vi "Test Coffee Shop Remove Customer Broadcast Name.vi"(8 "error in (no error)":errorcluster, 11 "Coffee Shop Test In":refnum<class "Coffee Shop Test.lvclass">) -> (0 "error out":errorcluster, 3 "Coffee Shop Test Out":refnum<class "Coffee Shop Test.lvclass">)   [LabVIEW 2020, in "Coffee Shop Test.lvclass"]
uses:
  Coffee Shop Test.lvclass
  Coffee Shop/Coffee Shop.lvclass
  <vilib>/Asteme/Triarc Framework/Process/Process.lvclass
  C:/Program Files (x86)/National Instruments/LabVIEW 2020/vi.lib/Asteme/Triarc Framework/Application/Application.lvclass
  C:/Program Files (x86)/National Instruments/LabVIEW 2020/vi.lib/Asteme/Triarc Framework/Process/Process.lvclass
  C:/Program Files (x86)/National Instruments/LabVIEW 2020/vi.lib/Asteme/Triarc Framework/Base/Base.lvclass
  C:/Program Files (x86)/National Instruments/LabVIEW 2020/vi.lib/Asteme/Triarc Framework/Error Handler Interface/Error Handler Interface.lvclass
  C:/Program Files (x86)/National Instruments/LabVIEW 2020/vi.lib/Asteme/Triarc Framework/Logging/Logging.lvclass
  C:/Users/anton/Documents/GitHub/Triarc-Examples/Coffee Shop/Coffee Shop/Coffee Shop.lvclass
  <vilib>/Asteme/Triarc Framework Test Suite/Support/Event Helpers/Event Helpers.lvlib
  <vilib>/Asteme/LUnit/Test Case.lvclass
  C:/Program Files (x86)/National Instruments/LabVIEW 2020/vi.lib/Asteme/Triarc Framework Test Suite/Application Test/Application Test.lvclass
  C:/Program Files (x86)/National Instruments/LabVIEW 2020/vi.lib/Asteme/Triarc Framework Test Suite/Process Test/Process Test.lvclass
  C:/Program Files (x86)/National Instruments/LabVIEW 2020/vi.lib/Asteme/Triarc Framework Test Suite/Base Class Test/Base Test.lvclass
  C:/Program Files (x86)/National Instruments/LabVIEW 2020/vi.lib/Asteme/LUnit/Test Case.lvclass
  C:/Users/anton/Documents/GitHub/Triarc-Examples/Coffee Shop/Coffee Shop Test/Coffee Shop Test.lvclass
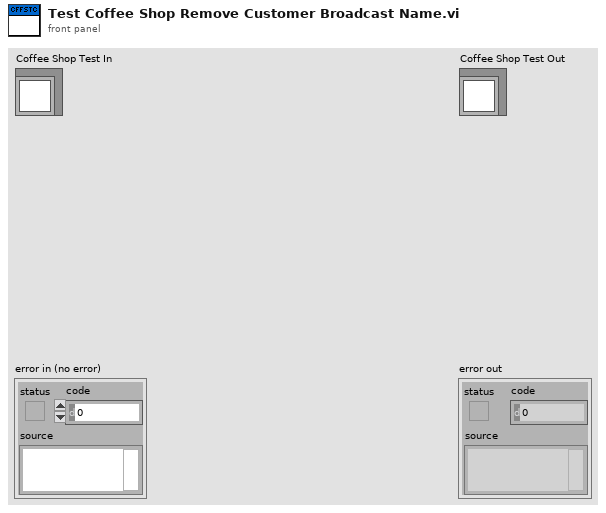
[diagram p1: front panel]
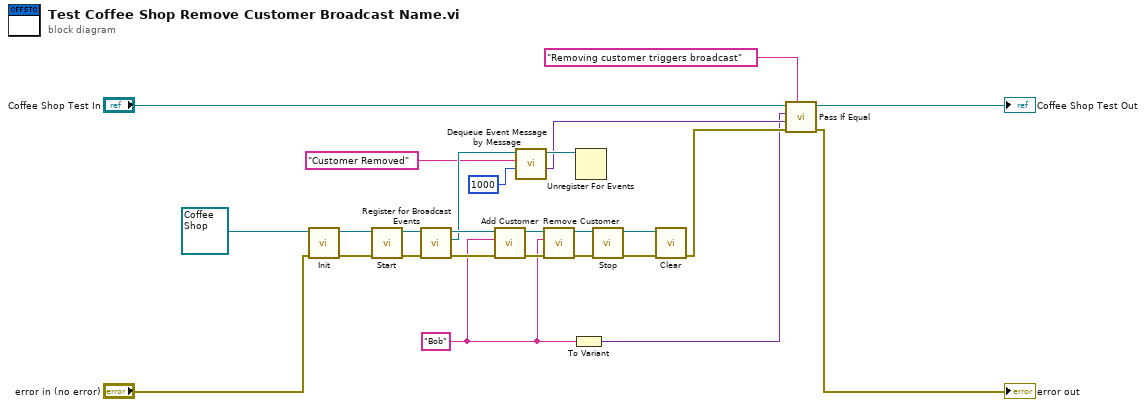
[diagram p0: block diagram]
diagram:
  w1 = "Bob" ("Name")
  n1 = call-dynamic "Init.vi"("error in (no error)"="error in (no error)", "Process In"=refnum<class "Coffee Shop.lvclass"> refnum ("Coffee Shop.lvclass")) -> ("error out"=w24:errorcluster, "Process Out"=w25:refnum<class "Coffee Shop.lvclass">)  [unwired: 8 in]
  n2 = call <vilib>:"Start.vi"("error in (no error)"=w24, "Process In"=w25) -> ("error out"=w23:errorcluster, "Process Out"=w17:refnum<class "Coffee Shop.lvclass">)  [unwired: 8 in]
  n3 = call <vilib>:"Register for Broadcast Events.vi"("error in (no error)"=w23, "Process In"=w17) -> ("error out"=w18:errorcluster, "Event Registration Refnum Out"=w15:refnum<event-registration>, "Process Out"=w16:refnum<class "Coffee Shop.lvclass">)  [unwired: 7 in]
  n4 = call "Add Customer.vi"("error in (no error)"=w18, "Name"=w1, "Coffee Shop in"=w16) -> ("error out"=w19:errorcluster, "Coffee Shop out"=w3:refnum<class "Coffee Shop.lvclass">)  [unwired: 7 in]
  n5 = call <vilib>:"Dequeue Event Message by Message.vi"("Timeout (-1)"=1000, "Message"="Customer Removed", "Event Registration Refnum"=w15) -> ("Message Data"=w6:variant, "Event Registration Refnum Out"=w13:refnum<event-registration>)  [unwired: 4 in, 3 out]
  n6 = call "Remove Customer.vi"("error in (no error)"=w19, "Name"=w1, "Coffee Shop In"=w3) -> ("error out"=w4:errorcluster, "Coffee Shop Out"=w2:refnum<class "Coffee Shop.lvclass">)  [unwired: 7 in]
  n7 = To Variant(anything=w1) -> (Variant=w5:variant)
  n8 = Unregister For Events(event registration refnum=w13) -> ()  [unwired: 1 in, 1 out]
  n9 = call <vilib>:"Stop.vi"("error in (no error)"=w4, "Process In"=w2) -> ("error out"=w21:errorcluster, "Process Out"=w22:refnum<class "Coffee Shop.lvclass">)  [unwired: 7 in, 1 out]
  n10 = call-dynamic "Clear.vi"("error in (no error)"=w21, "Application In"=w22) -> ("error out"=w9:errorcluster)  [unwired: 9 in]
  n11 = call <vilib>:"Pass If Equal.vi"("Description"="Removing customer triggers broadcast", "error in (no error)"=w9, "Actual"=w6, "Expected"=w5, "Test Case In"="Coffee Shop Test In") -> ("error out"=→"error out":errorcluster, "Test Case Out"=→"Coffee Shop Test Out":refnum<class "Coffee Shop Test.lvclass">)  [unwired: 5 in]
